vi "Formula Aliases Storage.vi"(4 "Sort":bool, 6 "Get (F)/Set":bool, 8 "Alias list modified since last saved":bool, 9 "Descriptions Array in":string[](array[string]), 10 "Definitions Array in":string[](array[string]), 11 "Aliases Array in":string[](array[string])) -> (0 "Alias list modified since last saved":bool, 1 "Descriptions Array":string[](array[string]), 2 "Definitions Array":string[](array[string]), 3 "Aliases Array":string[](array[string]))   [LabVIEW 2021, in "Formula.lvlib"]
uses:
  Formula.lvlib
  <userlib>/_OpenG.lib/array/array.llb/openg_array.lvlib
  <userlib>/_OpenG.lib/array/array.llb/Sort 1D Array (String)__ogtk.vi
  <userlib>/_OpenG.lib/array/array.llb/Reorder 1D Array2 (String)__ogtk.vi
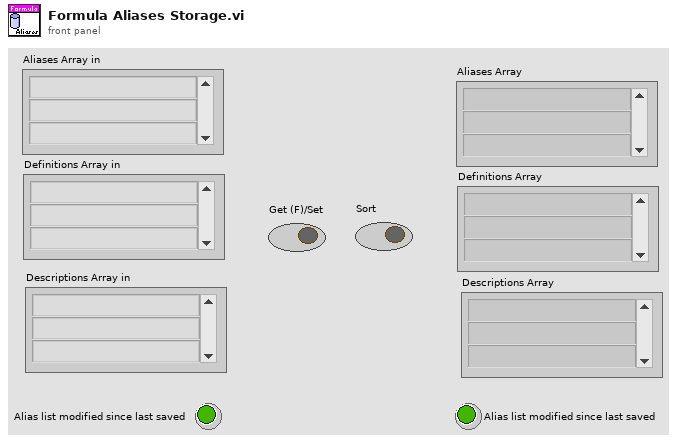
[diagram p1: front panel]
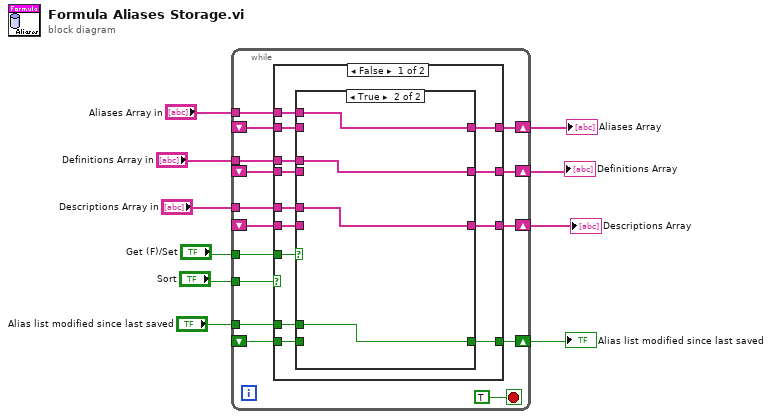
[diagram p0: block diagram]
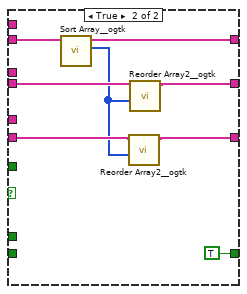
[diagram p3: hidden frame]
diagram:
  n1 = while {
    tunnel: "Get (F)/Set" -> [w24]
    shift-right: [w23] -> w7
    shift-left: _ -> [w22]
    shift-right: [w20] -> w6
    shift-left: _ -> [w18]
    tunnel: "Definitions Array in" -> [w21]
    tunnel: "Aliases Array in" -> [w19]
    tunnel: "Sort" -> [w17]
    shift-right: [w15] -> w3
    shift-left: _ -> [w14]
    tunnel: "Descriptions Array in" -> [w16]
    tunnel: "Alias list modified since last saved" -> [w13]
    shift-right: [w12] -> w1
    shift-left: _ -> [w11]
    stop <- TRUE stop-if-true
    n2 = case shown="False" w17 {
      tunnel: w24 -> [w38 _]
      tunnel: [w37 w53] -> w23
      tunnel: w22 -> [w36 w54]
      tunnel: w21 -> [w35 _]
      tunnel: [w34 w51] -> w20
      tunnel: w19 -> [w33 _]
      tunnel: w18 -> [w32 w52]
      tunnel: w16 -> [w30 _]
      tunnel: [w31 w48] -> w15
      tunnel: w14 -> [w29 w50]
      tunnel: w13 -> [w26 _]
      tunnel: [w27 TRUE ("Alias list modified since last saved 2")] -> w12
      tunnel: w11 -> [w28 _]
      frame False {
        n3 = case shown="True" w38 {
          tunnel: [w42 w45] -> w37
          tunnel: w36 -> [w42 _]
          tunnel: w35 -> [_ w46]
          tunnel: [w41 w46] -> w34
          tunnel: w33 -> [_ w45]
          tunnel: w32 -> [w41 _]
          tunnel: [w40 w44] -> w31
          tunnel: w30 -> [_ w44]
          tunnel: w29 -> [w40 _]
          tunnel: w28 -> [w39 _]
          tunnel: [w39 w43] -> w27
          tunnel: w26 -> [_ w43]
          frame False {
          }
          frame True {
          }
        }
      }
      frame True {
        n4 = call-poly <userlib>:"Sort Array__ogtk.vi"("Array in"=w54) -> ("Sorted Pointers"=w49:i32[], "Sorted Array out"=w53:string[])  [unwired: 9 in]
        n5 = call-poly <userlib>:"Reorder Array2__ogtk.vi"("indices"=w49, "array"=w50) -> ("reordered array"=w48:string[])  [unwired: 9 in]
        n6 = call-poly <userlib>:"Reorder Array2__ogtk.vi"("indices"=w49, "array"=w52) -> ("reordered array"=w51:string[])  [unwired: 9 in]
      }
    }
  }
  "Aliases Array" <- w7
  "Definitions Array" <- w6
  "Descriptions Array" <- w3
  "Alias list modified since last saved" <- w1
